vi "Post-Build Action.vi"(5 "Files Generated by Build":path[](array[path]), 6 "Top Level/Always Included VIs":path[](array[path]), 7 "Destination Path":path, 8 "error in (no error)":errorcluster, 9 "Target Name":string, 10 "Build Specification Name":string, 11 "Project Path":path) -> (0 "error out":errorcluster)   [LabVIEW 2020, in "ni-veristand-steps-runtime-lib.lvlib"]
uses:
  ni-veristand-steps-runtime-lib.lvlib
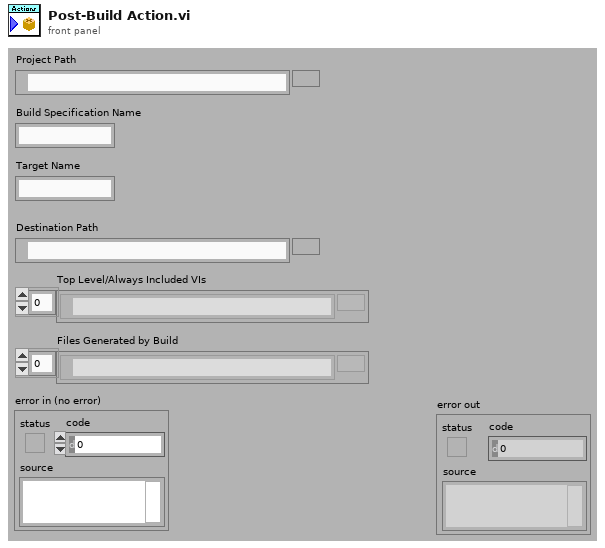
[diagram p1: front panel]
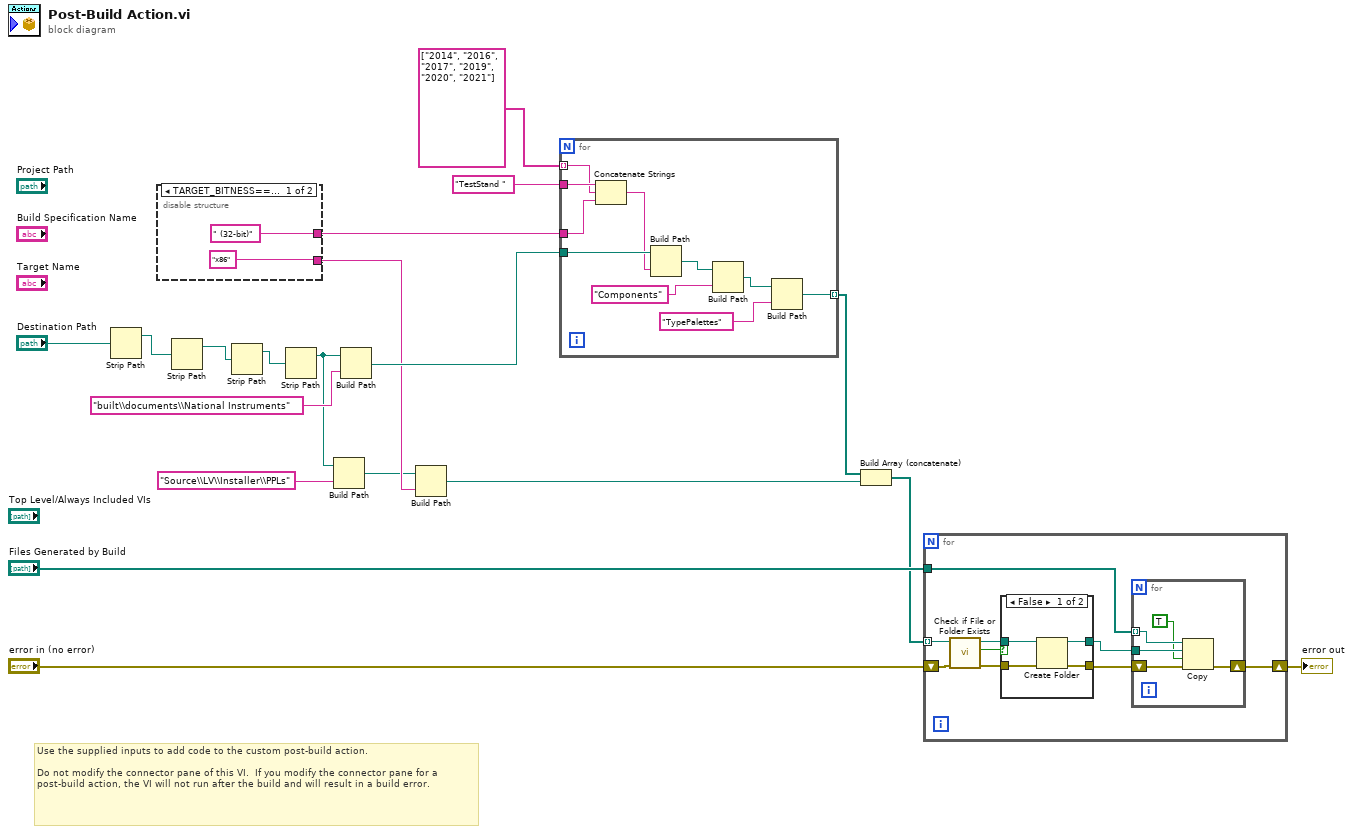
[diagram p0: block diagram]
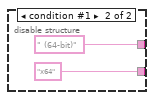
[diagram p3: hidden frame]
diagram:
  # "Use the supplied inputs to add code to the custom post-build action.\n\nDo not modify the connector pane of this VI.  If you modify the connector pane for a post-build action, the VI will not run after the build and will result in a build error."
  n1 = Strip Path(path="Destination Path") -> (stripped path=w15:path)  [unwired: 1 out]
  n2 = disable-structure shown="TARGET_BITNESS==32, Default" {
    disable-tunnel: [" (32-bit)" " (64-bit)"] -> w9
    disable-tunnel: ["x86" "x64"] -> w5
    frame condition #0 (active) {
    }
    frame condition #1 {
    }
  }
  n3 = Strip Path(path=w15) -> (stripped path=w14:path)  [unwired: 1 out]
  n4 = Strip Path(path=w14) -> (stripped path=w13:path)  [unwired: 1 out]
  n5 = Strip Path(path=w13) -> (stripped path=w7:path)  [unwired: 1 out]
  n6 = Build Path(base path=w7, name or relative path="Source\\LV\\Installer\\PPLs") -> (appended path=w4:path)
  n7 = Build Path(base path=w7, name or relative path="built\\documents\\National Instruments") -> (appended path=w8:path)
  n8 = Build Path(base path=w4, name or relative path=w5) -> (appended path=w2:path)
  n9 = for {
    tunnel: "TestStand " ("string") -> [w33]
    tunnel: string[] ["2014", "2016", "2017", "2019", "2020", "2021"] -> [w32] mode=indexing
    tunnel: w9 -> [w31]
    tunnel: w8 -> [w30]
    tunnel: [w24] -> w3 mode=indexing
    n10 = Concatenate Strings(w33, w32, w31) -> (w29:string)
    n11 = Build Path(base path=w30, name or relative path=w29) -> (appended path=w28:path)
    n12 = Build Path(base path=w28, name or relative path="Components") -> (appended path=w26:path)
    n13 = Build Path(base path=w26, name or relative path="TypePalettes") -> (appended path=w24:path)
  }
  n14 = Build Array (concatenate)(w3, w2) -> (w1:path[])
  n15 = for {
    tunnel: "Files Generated by Build" -> [w35]
    shift-right: [w37] -> w18
    shift-left: "error in (no error)" -> [w42]
    tunnel: w1 -> [w34] mode=indexing
    n16 = call <vilib>:"Check if File or Folder Exists.vi"("error in (no error)"=w42, "path"=w34) -> ("error out"=w41:errorcluster, "file or folder exists?"=w40:bool, "dup path"=w39:path)  [unwired: 7 in]
    n17 = case shown="False" w40 {
      tunnel: w41 -> [w51 w52]
      tunnel: w39 -> [w49 w53]
      tunnel: [w50 w52] -> w38
      tunnel: [w48 w53] -> w36
      frame False {
        n18 = Create Folder(path (use dialog)=w49, error in=w51) -> (created path=w48:path, error out=w50:errorcluster)  [unwired: 1 in, 1 out]
      }
      frame True {
      }
    }
    n19 = for {
      tunnel: w36 -> [w45]
      shift-right: [w46] -> w37
      shift-left: w38 -> [w47]
      tunnel: w35 -> [w44] mode=indexing
      n20 = Copy(8:w47, 9:TRUE ("overwrite (F)"), 10:w45, 11:w44) -> (0:w46:errorcluster)  [unwired: 1 in, 2 out]
    }
  }
  "error out" <- w18
